vi "Tx Ch FIFO State.vi"(9 "State":u32, 10 "Channel":u8, 11 "devId":i32) -> (1 "State out":u32, 2 "devId out":i32, 3 "function return":i32)   [LabVIEW 2013, in "CHR34XXX.lvlib"]
doc: "DLL BOOL __stdcall CHR34XXX_TxCh_SetMode(IN int devId,IN BYTE Channel,IN BYTE Mode); DLL BOOL __stdcall CHR34XXX_TxCh_SetPeriod(IN int devId,IN BYTE Channel,IN DWORD Period); DLL BOOL __stdcall CHR34XXX_TxCh_FIFOState(IN int devId,IN BYTE Channel,OUT DWORD *State);"
uses:
  CHR34XXX.lvlib
  CHR34XXX.dll
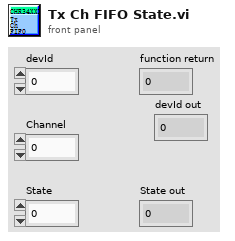
[diagram p1: front panel]
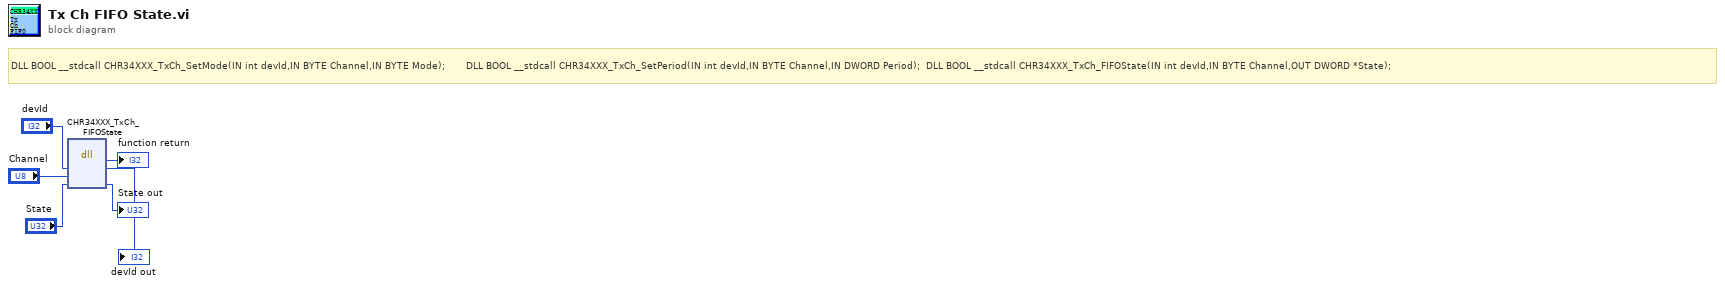
[diagram p0: block diagram]
diagram:
  # "DLL BOOL __stdcall CHR34XXX_TxCh_SetMode(IN int devId,IN BYTE Channel,IN BYTE Mode);       DLL BOOL __stdcall CHR34XXX_TxCh_SetPeriod(IN int devId,IN BYTE Channel,IN DWORD Period);  DLL BOOL __stdcall CHR34XXX_TxCh_FIFOState(IN int devId,IN BYTE Channel,OUT DWORD *State);"
  n1 = dll-call lib="C:/Users/Administrator/Desktop/CHR34XXX_lv/lv_lib/CHR34XXX.*" fn="CHR34XXX_TxCh_FIFOState"("devId"="devId", "Channel"="Channel", "State"="State") -> (→"function return":i32, "devId"=→"devId out":i32, "State"=→"State out":u32)  [unwired: 4 in, 2 out]
